vi "Color Sensors.vi"() -> ()   [LabVIEW 2020]
uses:
  <vilib>/Rock Robotics/SystemInterfaces/i2clib/i2c_bus.ctl
panel:
  in  "Blue Calibration":cluster{"R":dbl, "G":dbl, "B":dbl}={"R"=0.143, "G"=0.427, "B"=0.429}
  in  "Green Calibration":cluster{"R":dbl, "G":dbl, "B":dbl}={"R"=0.197, "G"=0.561, "B"=0.24}
  in  "Red Calibration":cluster{"R":dbl, "G":dbl, "B":dbl}={"R"=0.561, "G"=0.323, "B"=0.114}
  in  "Yellow Calibration":cluster{"R":dbl, "G":dbl, "B":dbl}={"R"=0.361, "G"=0.524, "B"=0.113}
  in  "I2C Bus":T1=enum."I2C MXP"
  out "Matched Color Name":string
  out "Match Confidence":dbl
  out "Measured Color":cluster{"R":dbl, "G":dbl, "B":dbl}
  out "error out":errorcluster
  out "Proximity":u16(graph)
  out "Color":u32(colorbox)
  in  "Finish":bool
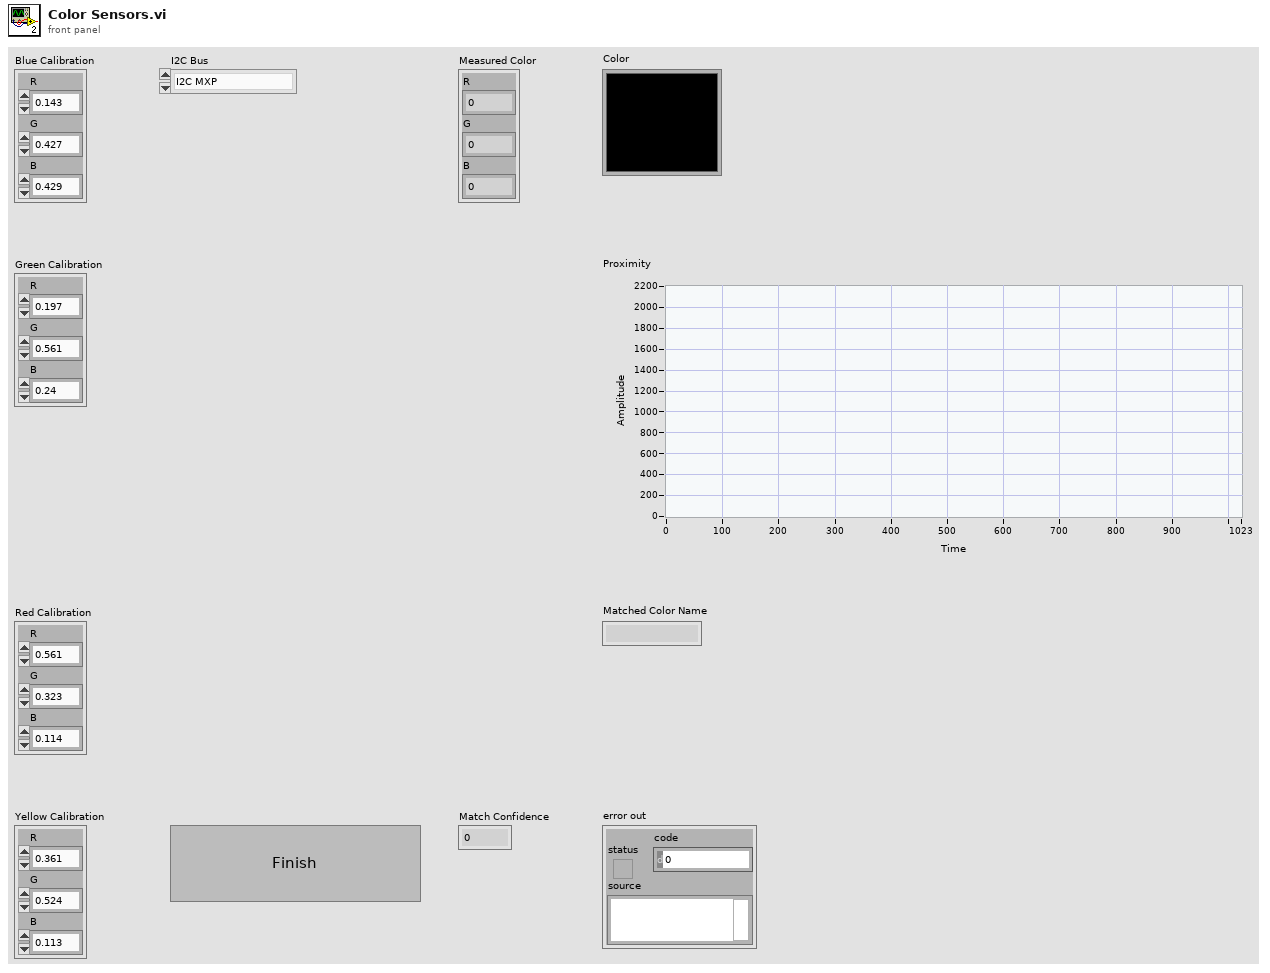
[diagram p1: front panel]
types:
  T1 = typedef "i2c_bus.ctl" = enum16{"I2C On-Board", "I2C MXP", "Invalid"}
  T2 = typedef "Color Sensor V3 DevRef.ctl" = cluster{"I2CDevRef":T3}
  T3 = typedef "WPI_I2CDevRef.ctl" = cluster{"DevStatus":errorcluster, "Device Address":u8, "Handle":i32, "I2C Bus":T1}
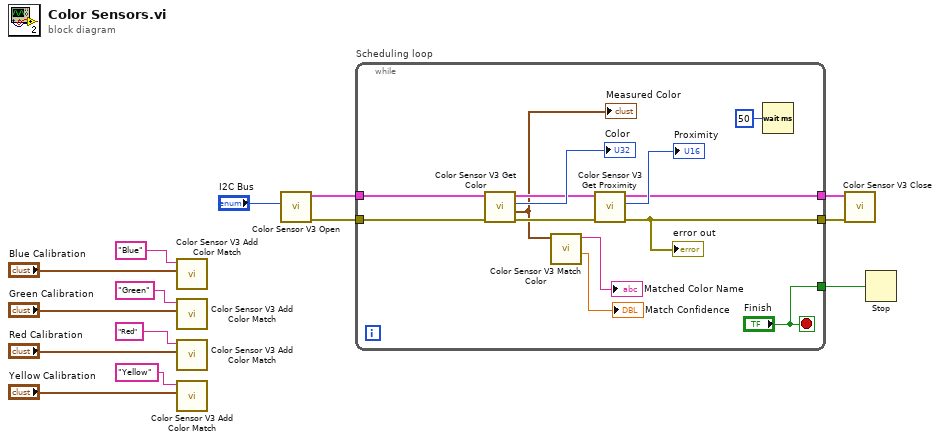
[diagram p0: block diagram]
diagram:
  n1 = call <vilib>:"Color Sensor V3 Add Color Match.vi"("Color"="Blue Calibration", "Name"="Blue") -> ()  [unwired: 10 in]
  n2 = call <vilib>:"Color Sensor V3 Add Color Match.vi"("Color"="Green Calibration", "Name"="Green") -> ()  [unwired: 10 in]
  n3 = call <vilib>:"Color Sensor V3 Add Color Match.vi"("Color"="Red Calibration", "Name"="Red") -> ()  [unwired: 10 in]
  n4 = call <vilib>:"Color Sensor V3 Add Color Match.vi"("Color"="Yellow Calibration", "Name"="Yellow") -> ()  [unwired: 10 in]
  n5 = call <vilib>:"Color Sensor V3 Open.vi"("I2C Bus"="I2C Bus") -> ("error out"=w3:errorcluster, "ColorSensorDevRef"=w2:T2)  [unwired: 9 in]
  n6 = while "Scheduling loop" {
    tunnel: w2 -> [w21]
    tunnel: w3 -> [w20]
    tunnel: ["Finish"] -> w4
    tunnel: [w16] -> w13
    tunnel: [w15] -> w14
    stop <- "Finish" stop-if-true
    n7 = call <vilib>:"Color Sensor V3 Get Color.vi"("error in (no error)"=w20, "ColorSensorDevRef"=w21) -> ("error out"=w25:errorcluster, "Normalized Color"=w19:cluster{"R":dbl, "G":dbl, "B":dbl}, "Color"=→"Color":u32, "ColorSensorDevRef out"=w24:T2)  [unwired: 6 in]
    "Measured Color" <- w19
    n8 = call <vilib>:"Color Sensor V3 Match Color.vi"("Measured Color"=w19) -> ("Confidence"=→"Match Confidence":dbl, "Matched Color Name"=→"Matched Color Name":string)  [unwired: 8 in, 1 out]
    n9 = call <vilib>:"Color Sensor V3 Get Proximity.vi"("error in (no error)"=w25, "ColorSensorDevRef"=w24) -> ("error out"=w15:errorcluster, "Proximity"=→"Proximity":u16, "ColorSensorDevRef out"=w16:T2)  [unwired: 7 in]
    "error out" <- w15
    n10 = Wait (ms)(milliseconds to wait=u32 50) -> ()  [unwired: 1 out]
  }
  n11 = call <vilib>:"Color Sensor V3 Close.vi"("error in (no error)"=w14, "ColorSensorDevRef in"=w13) -> ()  [unwired: 9 in, 1 out]
  n12 = Stop(stop? (T)=w4) -> ()
